vi "Close.vi"(8 "error in (no error)":errorcluster, 11 "Stream Download Controller in":refnum<class "Stream Download Controller.lvclass">) -> (0 "error out":errorcluster, 3 "Stream Download Controller out":refnum<class "Stream Download Controller.lvclass">)   [LabVIEW 2020, in "NI_SFTP.lvlib" / "Stream Download Controller.lvclass"]
uses:
  <vilib>/net/SFTP/API/Support/Download/Stream/Stream Download Controller.lvclass
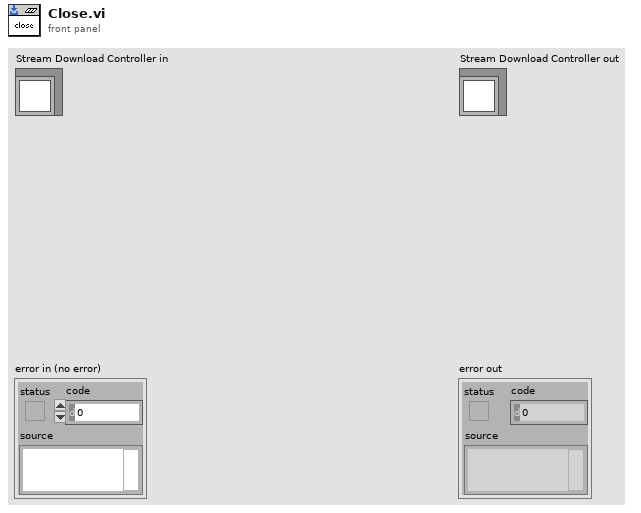
[diagram p1: front panel]
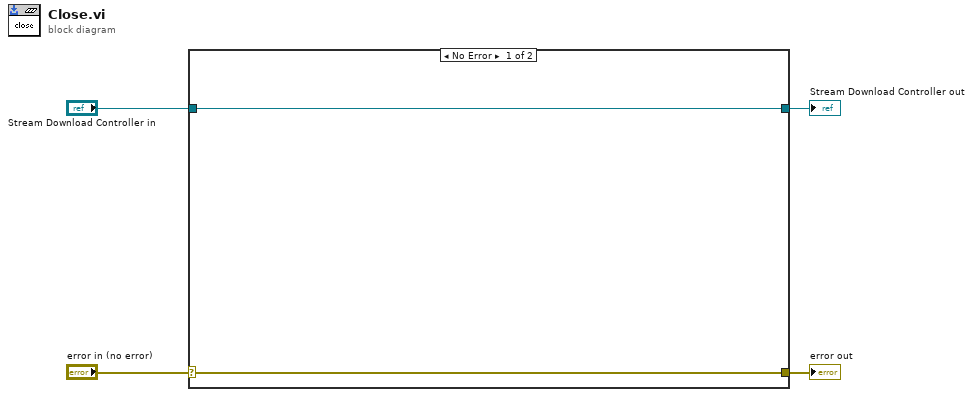
[diagram p0: block diagram]
diagram:
  n1 = case shown="No Error" "error in (no error)" {
    selector: "error in (no error)" -> [w6 w8]
    tunnel: [w6 w8] -> w3
    tunnel: [w5 w7] -> w1
    tunnel: "Stream Download Controller in" -> [w5 w7]
    frame No Error {
    }
    frame Error {
    }
  }
  "error out" <- w3
  "Stream Download Controller out" <- w1
